vi "Index to Key.vi"(11 "Index Out":i32) -> (3 "String":string)   [LabVIEW 2017, in "Futures.lvlib" / "Future.lvclass"]
uses:
  Future.lvclass
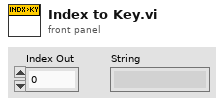
[diagram p1: front panel]
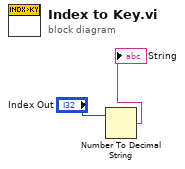
[diagram p0: block diagram]
diagram:
  n1 = Number To Decimal String(number="Index Out") -> (decimal integer string=→"String":string)  [unwired: 1 in]
